vi "gen MB frame -read Relay Status.vi"(11 "Dev Addr":u8=1 format="%x") -> (3 "MB frame":string)   [LabVIEW 2016, in "MB _relays.lvlib"]
uses:
  MB _relays.lvlib
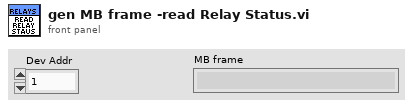
[diagram p1: front panel]
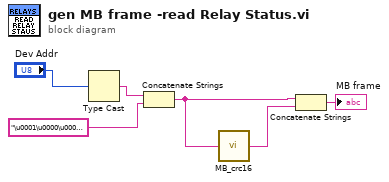
[diagram p0: block diagram]
diagram:
  n1 = Type Cast(x="Dev Addr") -> (*(type *) &x=w2:string)  [unwired: 1 in]
  n2 = Concatenate Strings(w2, "\u0001\u0000\u0000\u0000\b") -> (w1:string)
  n3 = call "MB_crc16.vi"("message"=w1) -> ("CRC16"=w6:string)  [unwired: 4 in]
  n4 = Concatenate Strings(w1, w6) -> (→"MB frame":string)
